vi "NI VeriStand - Get Item Root.vi"(8 "error in (no error)":errorcluster, 11 "Item Ref in":T1 format="%.0x") -> (0 "error out":errorcluster, 2 "Root Ref":T1 format="%.0x", 3 "Item Ref out":T1 format="%.0x", 4 "Found":bool)   [LabVIEW 2020, in "Custom Device Offline API.lvlib"]
uses:
  <vilib>/NI VeriStand/Custom Device Offline API/Custom Device Offline API.lvlib
  <vilib>/NI VeriStand/Custom Device API/Custom Device Item Ref.ctl
  NationalInstruments.VeriStand.SystemDefinitionAPI
  NationalInstruments.VeriStand.SystemStorage
  <vilib>/NI VeriStand/Custom Device API/Custom Device API.lvlib
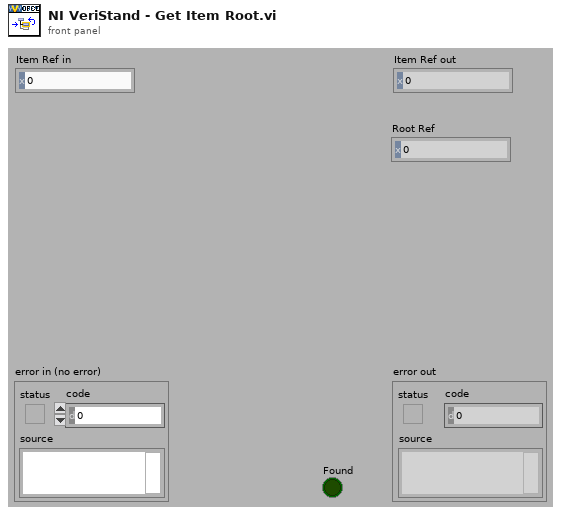
[diagram p1: front panel]
types:
  T1 = typedef "Custom Device API.lvlib/Custom Device Item Ref.ctl" = u64
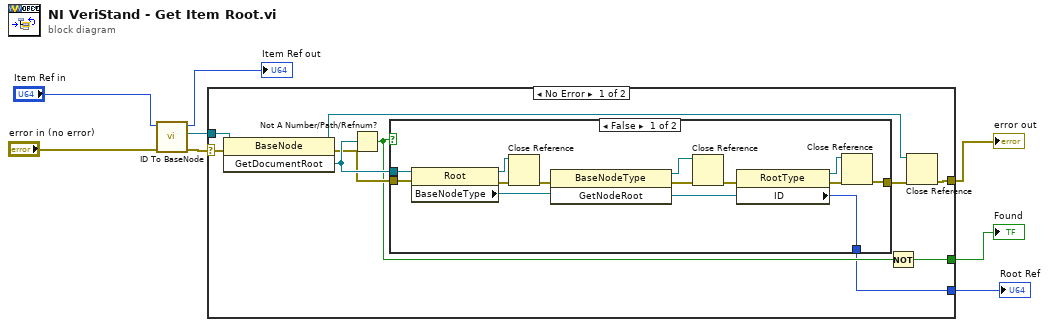
[diagram p0: block diagram]
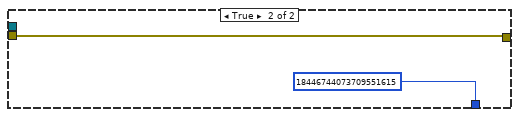
[diagram p2: hidden frame]
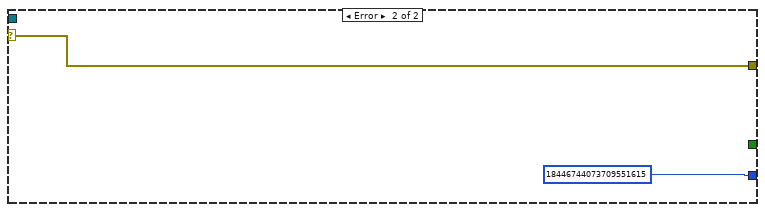
[diagram p3: hidden frame]
diagram:
  n1 = call <vilib>:"ID To BaseNode.vi"("error in (no error)"="error in (no error)", "ID in"="Item Ref in") -> ("error out"=w6:errorcluster, "BaseNode"=w4:refnum<k24>, "ID out"=→"Item Ref out":u64)  [unwired: 7 in]
  n2 = case shown="No Error" w6 {
    selector: w6 -> [w17 w36]
    tunnel: w4 -> [w18 _]
    tunnel: [w10 w36] -> w3
    tunnel: [w13 _] -> w2
    tunnel: [w12 T1 18446744073709551615 ("Parent Ref")] -> w1
    frame No Error {
      n3 = invoke class="BaseNode" method="GetDocumentRoot"(reference=w18, error in=w17) -> (reference out=w9:refnum<k24>, error out=w15:errorcluster, "GetDocumentRoot"=w16:refnum<k24>)  [unwired: 1 in]
      n4 = Not A Number/Path/Refnum?(number/path/refnum=w16) -> (NaN/Path/Refnum?=w14:bool)
      n5 = case shown="False" w14 {
        tunnel: [w20 w34] -> w11
        tunnel: w16 -> [w31 _]
        tunnel: w15 -> [w30 w34]
        tunnel: [w25 T1 18446744073709551615 ("Parent Ref")] -> w12
        frame False {
          n6 = property class="Root"(reference=w31, error in=w30) -> (reference out=w29:refnum<k24>, error out=w32:errorcluster, "BaseNodeType"=w27:refnum<k24>)
          n7 = Close Reference(reference=w29, error in (no error)=w32) -> (error out=w28:errorcluster)
          n8 = invoke class="BaseNodeType" method="GetNodeRoot"(reference=w27, error in=w28) -> (reference out=w24:refnum<k24>, error out=w23:errorcluster, "GetNodeRoot"=w26:refnum<k24>)  [unwired: 1 in]
          n9 = Close Reference(reference=w24, error in (no error)=w23) -> (error out=w19:errorcluster)
          n10 = property class="RootType"(reference=w26, error in=w19) -> (reference out=w21:refnum<k24>, error out=w22:errorcluster, "ID"=w25:u64)
          n11 = Close Reference(reference=w21, error in (no error)=w22) -> (error out=w20:errorcluster)
        }
        frame True {
        }
      }
      n12 = Not(x=w14) -> (.not. x?=w13:bool)
      n13 = Close Reference(reference=w9, error in (no error)=w11) -> (error out=w10:errorcluster)
    }
    frame Error {
    }
  }
  "error out" <- w3
  "Found" <- w2
  "Root Ref" <- w1
